vi "诊断标定4.vi"(8 "CAN端口":u16(ring), 9 "设备索引号":u16(ring), 10 "CAN卡类型":u32(ring)=4) -> ()   [LabVIEW 2013] (continued)
                n3552 = local read "设备索引号"() -> (w5173:u16)
                n3553 = local read "CAN卡类型"() -> (w5174:u32)
                n3554 = local read "CAN端口"() -> (w5172:u16)
                n3555 = call "标定授权发送.vi"("CAN卡类型"=w5174, "解锁类型"=enum16{"读取", "写", "下载"}."读取", "设备索引号"=w5173, "CAN端口"=w5172, "是否连接"=TRUE, "板选择"=0, "FUNC"=u32 1) -> ("发送成功"=w5179:bool)  [unwired: 8 out]
              }
            }
            n3556 = case shown="真" w5166 {
              tunnel: w5170 -> [w5181 w5186]
              tunnel: w5169 -> [w5180 w5185]
              tunnel: [w5181 w5183] -> w5168
              tunnel: [w5180 w5182] -> w5167
              frame False {
              }
              frame True {
                n3557 = Enqueue Element(queue=w5186, element="单个读取" ("元素"), error in (no error)=w5185) -> (queue out=w5183:refnum<queue>, error out=w5182:errorcluster)  [unwired: 2 out]
              }
            }
            n3558 = local write "写?"(FALSE ("写?")) -> ()
            n3559 = global write "EV05全局变量1.vi" "输出数组"(u8[] [] ("输出数组")) -> ()
            n3560 = call <vilib>:"Set Busy.vi"("disable click? (T)"=FALSE) -> ()  [unwired: 3 in, 8 out]
            n3561 = local write "清BUFF"(FALSE ("清BUFF")) -> ()
            n3562 = global write "EV05全局变量1.vi" "流控帧 2"(FALSE ("流控帧 2")) -> ()
            n3563 = local write "控制1"(TRUE ("控制1")) -> ()
            n3564 = local write "消除"(TRUE ("消除")) -> ()
          }
        }
      }
      event "全部读取": Value Change {
        n3565 = event-data() -> ("NewVal"=w5191:bool)  [unwired: 5 out]
        n3566 = case shown="真" w5191 {
          tunnel: w5190 -> [w5193 w5197]
          tunnel: w5189 -> [w5192 w5196]
          tunnel: [w5193 w5195] -> w5188
          tunnel: [w5192 w5194] -> w5187
          frame False {
          }
          frame True {
            n3567 = stacked-sequence {
              seq-local: [w5201 _] -> [_ _]
              seq-local: [w5200 _] -> [_ _]
              tunnel: w5197 -> [w5203 w5233]
              tunnel: w5196 -> [w5202 w5232]
              tunnel: [_ w5243] -> w5195
              tunnel: [_ w5242] -> w5194
              frame #0 {
                n3568 = local read "路径"() -> (w5199:path)
                n3569 = Empty String/Path?(string/path=w5199) -> (empty?=w5198:bool)
                n3570 = case shown="假" w5198 {
                  tunnel: w5203 -> [w5212 w5230]
                  tunnel: w5202 -> [w5211 w5229]
                  tunnel: [w5207 w5229] -> w5201
                  tunnel: [w5206 w5230] -> w5200
                  frame False {
                    n3571 = global read "EV05全局变量1.vi" "授权功能"() -> (w5209:bool)
                    n3572 = case shown="假" w5209 {
                      tunnel: [TRUE ("发送成功") w5221] -> w5210
                      frame False {
                      }
                      frame True {
                        n3573 = local read "设备索引号"() -> (w5215:u16)
                        n3574 = local read "CAN卡类型"() -> (w5216:u32)
                        n3575 = local read "CAN端口"() -> (w5214:u16)
                        n3576 = call "标定授权发送.vi"("CAN卡类型"=w5216, "解锁类型"=enum16{"读取", "写", "下载"}."读取", "设备索引号"=w5215, "CAN端口"=w5214, "是否连接"=TRUE, "板选择"=0, "FUNC"=u32 1) -> ("发送成功"=w5221:bool)  [unwired: 8 out]
                      }
                    }
                    n3577 = case shown="真" w5210 {
                      tunnel: w5212 -> [w5223 w5228]
                      tunnel: w5211 -> [w5222 w5227]
                      tunnel: [w5223 w5225] -> w5206
                      tunnel: [w5222 w5224] -> w5207
                      frame False {
                      }
                      frame True {
                        n3578 = Enqueue Element(queue=w5228, element="读配置文件" ("元素"), error in (no error)=w5227) -> (queue out=w5225:refnum<queue>, error out=w5224:errorcluster)  [unwired: 2 out]
                      }
                    }
                    n3579 = call <vilib>:"Set Busy.vi"("disable click? (T)"=FALSE) -> ()  [unwired: 3 in, 8 out]
                    n3580 = local write "布尔"(FALSE ("布尔")) -> ()
                    n3581 = Wait Until Next ms Multiple(millisecond multiple=u32 200 ("毫秒倍数")) -> ()  [unwired: 1 out]
                  }
                  frame True {
                  }
                }
              }
              frame #1 {
                n3582 = global read "EV05全局变量1.vi" "授权功能"() -> (w5236:bool)
                n3583 = case shown="假" w5236 {
                  tunnel: [TRUE ("发送成功") w5252] -> w5241
                  frame False {
                  }
                  frame True {
                    n3584 = local read "设备索引号"() -> (w5246:u16)
                    n3585 = local read "CAN卡类型"() -> (w5247:u32)
                    n3586 = local read "CAN端口"() -> (w5245:u16)
                    n3587 = call "标定授权发送.vi"("CAN卡类型"=w5247, "解锁类型"=enum16{"读取", "写", "下载"}."读取", "设备索引号"=w5246, "CAN端口"=w5245, "是否连接"=TRUE, "板选择"=0, "FUNC"=u32 1) -> ("发送成功"=w5252:bool)  [unwired: 8 out]
                  }
                }
                n3588 = local write "写?"(FALSE ("写?")) -> ()
                n3589 = call <vilib>:"Set Busy.vi"("disable click? (T)"=FALSE) -> ()  [unwired: 3 in, 8 out]
                n3590 = global write "EV05全局变量1.vi" "输出数组"(u8[] [] ("输出数组")) -> ()
                n3591 = global write "EV05全局变量1.vi" "流控帧 2"(FALSE ("流控帧 2")) -> ()
                n3592 = case shown="真" w5241 {
                  tunnel: w5233 -> [w5254 w5259]
                  tunnel: w5232 -> [w5253 w5258]
                  tunnel: [w5254 w5256] -> w5243
                  tunnel: [w5253 w5255] -> w5242
                  frame False {
                  }
                  frame True {
                    n3593 = Enqueue Element(queue=w5259, element="全部读取" ("元素"), error in (no error)=w5258) -> (queue out=w5256:refnum<queue>, error out=w5255:errorcluster)  [unwired: 2 out]
                  }
                }
                n3594 = local write "清BUFF"(FALSE ("清BUFF")) -> ()
                n3595 = local write "控制1"(TRUE ("控制1")) -> ()
                n3596 = local write "消除"(TRUE ("消除")) -> ()
              }
            }
          }
        }
      }
      event "开启均衡": Value Change {
        n3597 = event-data() -> ("NewVal"=w5264:bool)  [unwired: 5 out]
        n3598 = case shown="真" w5264 {
          tunnel: w5263 -> [w5266 w5278]
          tunnel: w5262 -> [w5265 w5277]
          tunnel: [w5266 w5276] -> w5261
          tunnel: [w5265 w5275] -> w5260
          frame False {
          }
          frame True {
            n3599 = global read "EV05全局变量1.vi" "授权功能"() -> (w5270:bool)
            n3600 = case shown="假" w5270 {
              tunnel: [TRUE ("发送成功") w5288] -> w5274
              frame False {
              }
              frame True {
                n3601 = local read "主从选择"() -> (w5280:enum32{"主板", "从板"})
                n3602 = case shown="\"从板\"" w5280 {
                  tunnel: [0.0 ("FUNC") w5290] -> w5281
                  frame "主板", Default {
                  }
                  frame "从板" {
                    n3603 = local read "从板板号"() -> (w5290:u8)
                  }
                }
                n3604 = local read "设备索引号"() -> (w5283:u16)
                n3605 = local read "CAN卡类型"() -> (w5284:u32)
                n3606 = local read "CAN端口"() -> (w5282:u16)
                n3607 = call "标定授权发送.vi"("CAN卡类型"=w5284, "解锁类型"=enum16{"读取", "写", "下载"}."写", "设备索引号"=w5283, "CAN端口"=w5282, "是否连接"=TRUE, "板选择"=0, "FUNC"=w5281) -> ("发送成功"=w5288:bool)  [unwired: 8 out]
              }
            }
            n3608 = case shown="真" w5274 {
              tunnel: w5278 -> [w5292 w5297]
              tunnel: w5277 -> [w5291 w5296]
              tunnel: [w5292 w5294] -> w5276
              tunnel: [w5291 w5293] -> w5275
              frame False {
              }
              frame True {
                n3609 = Enqueue Element(queue=w5297, element="开启均衡" ("元素"), error in (no error)=w5296) -> (queue out=w5294:refnum<queue>, error out=w5293:errorcluster)  [unwired: 2 out]
              }
            }
            n3610 = local write "写?"(TRUE ("写?")) -> ()
            n3611 = local write "清BUFF"(FALSE ("清BUFF")) -> ()
            n3612 = local write "控制1"(TRUE ("控制1")) -> ()
            n3613 = global write "EV05全局变量1.vi" "流控帧 2"(FALSE ("流控帧 2")) -> ()
            n3614 = local write "消除"(TRUE ("消除")) -> ()
            n3615 = call <vilib>:"Set Busy.vi"("disable click? (T)"=TRUE) -> ()  [unwired: 3 in, 8 out]
          }
        }
      }
      event "关闭均衡": Value Change {
        n3616 = event-data() -> ("NewVal"=w5302:bool)  [unwired: 5 out]
        n3617 = case shown="真" w5302 {
          tunnel: w5301 -> [w5304 w5316]
          tunnel: w5300 -> [w5303 w5315]
          tunnel: [w5304 w5314] -> w5299
          tunnel: [w5303 w5313] -> w5298
          frame False {
          }
          frame True {
            n3618 = global read "EV05全局变量1.vi" "授权功能"() -> (w5308:bool)
            n3619 = case shown="假" w5308 {
              tunnel: [TRUE ("发送成功") w5326] -> w5312
              frame False {
              }
              frame True {
                n3620 = local read "主从选择"() -> (w5318:enum32{"主板", "从板"})
                n3621 = case shown="\"从板\"" w5318 {
                  tunnel: [0.0 ("FUNC") w5328] -> w5319
                  frame "主板", Default {
                  }
                  frame "从板" {
                    n3622 = local read "从板板号"() -> (w5328:u8)
                  }
                }
                n3623 = local read "设备索引号"() -> (w5321:u16)
                n3624 = local read "CAN卡类型"() -> (w5322:u32)
                n3625 = local read "CAN端口"() -> (w5320:u16)
                n3626 = call "标定授权发送.vi"("CAN卡类型"=w5322, "解锁类型"=enum16{"读取", "写", "下载"}."写", "设备索引号"=w5321, "CAN端口"=w5320, "是否连接"=TRUE, "板选择"=0, "FUNC"=w5319) -> ("发送成功"=w5326:bool)  [unwired: 8 out]
              }
            }
            n3627 = case shown="真" w5312 {
              tunnel: w5316 -> [w5330 w5335]
              tunnel: w5315 -> [w5329 w5334]
              tunnel: [w5330 w5332] -> w5314
              tunnel: [w5329 w5331] -> w5313
              frame False {
              }
              frame True {
                n3628 = Enqueue Element(queue=w5335, element="关闭均衡" ("元素"), error in (no error)=w5334) -> (queue out=w5332:refnum<queue>, error out=w5331:errorcluster)  [unwired: 2 out]
              }
            }
            n3629 = local write "写?"(TRUE ("写?")) -> ()
            n3630 = local write "清BUFF"(FALSE ("清BUFF")) -> ()
            n3631 = local write "控制1"(TRUE ("控制1")) -> ()
            n3632 = global write "EV05全局变量1.vi" "流控帧 2"(FALSE ("流控帧 2")) -> ()
            n3633 = local write "消除"(TRUE ("消除")) -> ()
            n3634 = call <vilib>:"Set Busy.vi"("disable click? (T)"=TRUE) -> ()  [unwired: 3 in, 8 out]
          }
        }
      }
      event "强制开启均衡": Value Change {
        n3635 = event-data() -> ("NewVal"=w5340:bool)  [unwired: 5 out]
        n3636 = case shown="真" w5340 {
          tunnel: w5339 -> [w5342 w5354]
          tunnel: w5338 -> [w5341 w5353]
          tunnel: [w5342 w5352] -> w5337
          tunnel: [w5341 w5351] -> w5336
          frame False {
          }
          frame True {
            n3637 = global read "EV05全局变量1.vi" "授权功能"() -> (w5346:bool)
            n3638 = case shown="假" w5346 {
              tunnel: [TRUE ("发送成功") w5364] -> w5350
              frame False {
              }
              frame True {
                n3639 = local read "主从选择"() -> (w5356:enum32{"主板", "从板"})
                n3640 = case shown="\"从板\"" w5356 {
                  tunnel: [0.0 ("FUNC") w5366] -> w5357
                  frame "主板", Default {
                  }
                  frame "从板" {
                    n3641 = local read "从板板号"() -> (w5366:u8)
                  }
                }
                n3642 = local read "设备索引号"() -> (w5359:u16)
                n3643 = local read "CAN卡类型"() -> (w5360:u32)
                n3644 = local read "CAN端口"() -> (w5358:u16)
                n3645 = call "标定授权发送.vi"("CAN卡类型"=w5360, "解锁类型"=enum16{"读取", "写", "下载"}."写", "设备索引号"=w5359, "CAN端口"=w5358, "是否连接"=TRUE, "板选择"=0, "FUNC"=w5357) -> ("发送成功"=w5364:bool)  [unwired: 8 out]
              }
            }
            n3646 = case shown="真" w5350 {
              tunnel: w5354 -> [w5368 w5373]
              tunnel: w5353 -> [w5367 w5372]
              tunnel: [w5368 w5370] -> w5352
              tunnel: [w5367 w5369] -> w5351
              frame False {
              }
              frame True {
                n3647 = Enqueue Element(queue=w5373, element="强制均衡" ("元素"), error in (no error)=w5372) -> (queue out=w5370:refnum<queue>, error out=w5369:errorcluster)  [unwired: 2 out]
              }
            }
            n3648 = local write "写?"(TRUE ("写?")) -> ()
            n3649 = local write "清BUFF"(FALSE ("清BUFF")) -> ()
            n3650 = local write "控制1"(TRUE ("控制1")) -> ()
            n3651 = global write "EV05全局变量1.vi" "流控帧 2"(FALSE ("流控帧 2")) -> ()
            n3652 = local write "消除"(TRUE ("消除")) -> ()
            n3653 = call <vilib>:"Set Busy.vi"("disable click? (T)"=TRUE) -> ()  [unwired: 3 in, 8 out]
          }
        }
      }
    }
    n3654 = Unbundle By Name(w2868) -> ("status"=w2867:bool)
    n3655 = Or(x=w2867, y=w2869) -> (x .or. y?=w2870:bool)
  }
  n3656 = while {
    stop <- w5374 stop-if-true
    n3657 = local read "停止"() -> (w5374:bool)
    n3658 = local read "数据读取判定"() -> (w5375:bool)
    n3659 = case shown="真" w5375 {
      frame False {
        n3660 = Wait Until Next ms Multiple(millisecond multiple=u32 50 ("毫秒倍数")) -> ()  [unwired: 1 out]
      }
      frame True {
        n3661 = stacked-sequence {
          frame #0 {
            n3662 = Wait Until Next ms Multiple(millisecond multiple=u32 200 ("毫秒倍数")) -> ()  [unwired: 1 out]
          }
          frame #1 {
            n3663 = local read "临时"() -> (w5381:T1)
            n3664 = Add(x=2, y="循环") -> (x+y=w5379:i32)
            n3665 = for {
              N: w5379 -> [_]
              tunnel: w5381 -> [w5382] mode=indexing
              n3666 = local read "主从选择"() -> (w5383:enum32{"主板", "从板"})
              n3667 = local read "设备索引号"() -> (w5386:u16)
              n3668 = case shown="\"从板\"" w5383 {
                tunnel: [0 ("FUNC") w5392] -> w5384
                frame "主板", Default {
                }
                frame "从板" {
                  n3669 = local read "从板板号"() -> (w5392:u8)
                }
              }
              n3670 = local read "CAN卡类型"() -> (w5385:u32)
              n3671 = local read "CAN端口"() -> (w5387:u16)
              n3672 = local read "选项卡控件 2"() -> (w5390:T6)
              n3673 = disable-structure shown="禁用" {
                disable-tunnel: w5382 -> [w5393 _]
                frame Disabled {
                  n3674 = call "标定授权读取.vi"("VCI_Receive"=w5393) -> ()  [unwired: 1 out]
                }
                frame Enabled {
                }
              }
              n3675 = case shown="\"读写参数\", 默认" w5390 {
                tunnel: "写?" -> [w5400 _ _ _]
                tunnel: "命令" -> [w5401 w5497 w5754 w5886]
                tunnel: w5383 -> [w5408 _ w5760 w5892]
                tunnel: w5382 -> [_ _ _ _]
                tunnel: w5382 -> [w5394 w5488 w5748 w5877]
                tunnel: w5387 -> [w5405 w5498 w5756 w5888]
                tunnel: w5386 -> [w5404 w5499 w5757 w5889]
                tunnel: w5385 -> [w5403 w5500 w5758 w5890]
                tunnel: w5384 -> [w5402 _ w5755 w5887]
                frame "读写参数", Default {
                  n3676 = local read "命令序号"() -> (w5399:u8)
                  n3677 = call "多帧接收机制(EV05).vi"("can卡类型"=w5403, "设备索引号"=w5404, "CAN端口"=w5405, "VCI_Receive"=w5394, "命令"=w5401, "板号"=w5402, "写?"=w5400, "命令序号"=w5399) -> ("错误信号"=w5397:bool, "错误代码"=w5407:i32, "输出数组"=w5406:u8[], "读错误代码"=w5398:u8[], "结束信号"=w5395:bool)  [unwired: 7 out]
                  n3678 = local write "数据读取判定"(FALSE ("数据读取判定")) -> ()
                  n3679 = case shown="假" w5400 {
                    tunnel: w5395 -> [w5418 w5478]
                    tunnel: w5407 -> [w5417 w5477]
                    tunnel: w5399 -> [w5416 _]
                    tunnel: w5406 -> [w5415 _]
                    tunnel: w5401 -> [w5414 _]
                    tunnel: w5408 -> [w5411 w5476]
                    tunnel: w5398 -> [w5410 _]
                    tunnel: w5397 -> [w5409 _]
                    frame False {
                      # "读参数"
                      n3680 = local read "控制1"() -> (w5412:bool)
                      n3681 = And(x=w5412, y=w5418) -> (x .and. y?=w5413:bool)
                      n3682 = case shown="真" w5413 {
                        tunnel: w5417 -> [_ w5428]
                        tunnel: w5416 -> [_ w5427]
                        tunnel: w5415 -> [_ w5426]
                        tunnel: w5414 -> [_ w5425]
                        tunnel: w5411 -> [_ w5422]
                        tunnel: w5410 -> [_ w5420]
                        tunnel: w5409 -> [_ w5421]
                        frame False {
                        }
                        frame True {
                          n3683 = case shown="假" w5421 {
                            tunnel: w5428 -> [w5437 _]
                            tunnel: w5427 -> [w5436 _]
                            tunnel: w5426 -> [w5435 _]
                            tunnel: w5425 -> [w5433 _]
                            tunnel: w5422 -> [w5429 _]
                            tunnel: w5420 -> [_ w5462]
                            frame False {
                              n3684 = case shown="\"主板\", 默认" w5429 {
                                tunnel: [w5438 _] -> w5432
                                tunnel: [_ w5451] -> w5431
                                frame "主板", Default {
                                n3685 = stacked-sequence {
                                tunnel: [_ w5450] -> w5438
                                frame #0 {
                                n3686 = control-ref of="一级故障"() -> (w5444:refnum<vi>)
                                n3687 = control-ref of="一级故障 2"() -> (w5446:refnum<vi>)
                                n3688 = control-ref of="一级故障 3"() -> (w5447:refnum<vi>)
                                n3689 = control-ref of="加热控制参数"() -> (w5448:refnum<vi>)
                                n3690 = control-ref of="充电控制参数"() -> (w5449:refnum<vi>)
                                n3691 = control-ref of="电池信息"() -> (w5442:refnum<vi>)
                                n3692 = control-ref of="项目信息"() -> (w5445:refnum<vi>)
                                n3693 = control-ref of="一级故障 4"() -> (w5443:refnum<vi>)
                                n3694 = control-ref of="高压参数"() -> (w5441:refnum<vi>)
                                n3695 = local read "主板数据"() -> (w5440:T4)
                                n3696 = Bundle(cluster=w5440, "项目信息"=w5445, "一级故障 4"=w5443, "一级故障"=w5444, "一级故障 2"=w5446, "一级故障 3"=w5447, "加热控制参数"=w5448, "充电控制参数"=w5449, "高压参数"=w5441, "电池信息"=w5442) -> (w5439:T4)
                                n3697 = local write "主板数据"(w5439) -> ()
                                }
                                frame #1 {
                                n3698 = control-ref of="主板数据"() -> (w5450:refnum<vi>)
                                }
                                }
                                }
                                frame "从板" {
                                n3699 = stacked-sequence {
                                tunnel: [_ w5461] -> w5451
                                frame #0 {
                                n3700 = control-ref of="从板板号"() -> (w5454:refnum<vi>)
                                n3701 = control-ref of="项目信息 2"() -> (w5455:refnum<vi>)
                                n3702 = control-ref of="加热控制参数"() -> (w5456:refnum<vi>)
                                n3703 = control-ref of="一级故障(从板)"() -> (w5457:refnum<vi>)
                                n3704 = control-ref of="二级故障(从板)"() -> (w5458:refnum<vi>)
                                n3705 = control-ref of="三级故障(从板)"() -> (w5459:refnum<vi>)
                                n3706 = control-ref of="电池组信息(从板)"() -> (w5460:refnum<vi>)
                                n3707 = local read "从板数据"() -> (w5453:T3)
                                n3708 = Bundle(cluster=w5453, "从板板号"=w5454, "项目信息 2"=w5455, "加热控制参数"=w5456, "一级故障(从板)"=w5457, "二级故障(从板)"=w5458, "三级故障(从板)"=w5459, "电池组信息(从板)"=w5460) -> (w5452:T3)
                                n3709 = local write "从板数据"(w5452) -> ()
                                }
                                frame #1 {
                                n3710 = control-ref of="从板数据"() -> (w5461:refnum<vi>)
                                }
                                }
                                }
                              }
                              n3711 = control-ref of="结果"() -> (w5434:refnum<vi>)
                              n3712 = control-ref of="从板个数"() -> (w5430:refnum<vi>)
                              n3713 = call "输出数据解析.vi"("主板引用"=w5432, "从板引用"=w5431, "板选择"=w5429, "错误代码"=w5437, "命令序号"=w5436, "输入数组"=w5435, "命令"=w5433, "进度引用"=w5434, "从板个数"=w5430) -> ()  [unwired: 7 out]
                            }
                            frame True {
                              n3714 = Index Array(array=w5462, index #1=0 ("索引"), index #2=1 ("索引")) -> (element #1=w5465:u8, element #2=w5466:u8)
                              n3715 = Join Numbers(hi=w5465, lo=w5466) -> ((hi.lo)=w5464:u16)
                              n3716 = Number To Hexadecimal String(2:w5464) -> (0:w5463:string)  [unwired: 1 out]
                              n3717 = control-ref of="结果"() -> (w5471:refnum<vi>)
                              n3718 = Concatenate Strings("0x" ("字符串"), w5463) -> (w5472:string)
                              n3719 = Build Array(w5472) -> (w5473:string[])
                              n3720 = call "表格编辑.vi"("新元素/子数组"=w5473, "活动单元格:单元格背景色"=u32 16740749, "MCListbox引用句柄"=w5471) -> ()  [unwired: 9 out]
                            }
                          }
                          n3721 = global write "EV05全局变量1.vi" "流控帧 2"(FALSE ("流控帧 2")) -> ()
                          n3722 = local write "消除"(FALSE ("消除")) -> ()
                          n3723 = local write "控制1"(FALSE ("控制1")) -> ()
                        }
                      }
                    }
                    frame True {
                      # "写参数判定"
                      n3724 = And(x="控制1", y=w5478) -> (x .and. y?=w5475:bool)
                      n3725 = case shown="真" w5475 {
                        tunnel: w5477 -> [_ w5485]
                        tunnel: w5476 -> [_ w5482]
                        frame False {
                        }
                        frame True {
                          n3726 = call <vilib>:"Unset Busy.vi"() -> ()  [unwired: 2 in, 10 out]
                          n3727 = case shown="\"主板\", 默认" w5482 {
                            tunnel: [w5486 w5487] -> w5484
                            frame "主板", Default {
                              n3728 = local read "主板选项"() -> (w5486:string)
                            }
                            frame "从板" {
                              n3729 = local read "从板选项"() -> (w5487:string)
                            }
                          }
                          n3730 = control-ref of="结果"() -> (w5483:refnum<vi>)
                          n3731 = call "输入数据判定.vi"("主从选择"=w5482, "主板选项"=w5484, "进度引用"=w5483, "错误代码"=w5485) -> ()  [unwired: 2 in, 6 out]
                          n3732 = global write "EV05全局变量1.vi" "流控帧 2"(FALSE ("流控帧 2")) -> ()
                          n3733 = local write "控制1"(FALSE ("控制1")) -> ()
                          n3734 = local write "消除"(FALSE ("消除")) -> ()
                        }
                      }
                    }
                  }
                }
                frame "版本读取" {
                  n3735 = local read "命令序号"() -> (w5491:u8)
                  n3736 = local read "从板板号"() -> (w5494:u8)
                  n3737 = local read "控制1"() -> (w5495:bool)
                  n3738 = call "多帧接收机制(EV05).vi"("can卡类型"=w5500, "设备索引号"=w5499, "CAN端口"=w5498, "VCI_Receive"=w5488, "命令"=w5497, "板号"=w5494, "命令序号"=w5491) -> ("错误信号"=w5492:bool, "输出数组"=w5501:u8[], "读错误代码"=w5493:u8[], "结束信号"=w5489:bool)  [unwired: 1 in, 8 out]
                  n3739 = And(x=w5495, y=w5489) -> (x .and. y?=w5496:bool)
                  n3740 = case shown="真" w5496 {
                    tunnel: w5501 -> [_ w5509]
                    tunnel: w5491 -> [_ w5508]
                    tunnel: w5497 -> [_ w5507]
                    tunnel: w5493 -> [_ w5503]
                    tunnel: w5492 -> [_ w5502]
                    frame False {
                    }
                    frame True {
                      n3741 = case shown="假" w5502 {
                        tunnel: w5509 -> [w5513 _]
                        tunnel: w5508 -> [w5512 _]
                        tunnel: w5507 -> [w5511 _]
                        tunnel: w5503 -> [w5510 w5737]
                        frame False {
                          n3742 = case shown="89" w5511 {
                            tunnel: w5512 -> [_ w5516]
                            tunnel: w5513 -> [_ w5515]
                            tunnel: w5510 -> [_ _]
                            frame 0, Default {
                            }
                            frame 137 {
                              n3743 = case shown="1" w5516 {
                                tunnel: w5515 -> [_ w5544 w5588 w5608 w5735]
                                frame 0, Default {
                                }
                                frame 1 {
                                w5526 = "." ("字符串")
                                n3744 = Array Subset(array=w5544, index=0 ("索引"), length=14 ("长度")) -> (w5557:u8[])
                                n3745 = Index Array(array=w5544, index=14 ("索引")) -> (element=w5547:u8)
                                n3746 = Index Array(array=w5544, index #1=15 ("索引"), index #2=16 ("索引")) -> (element #1=w5553:u8, element #2=w5554:u8)
                                n3747 = Index Array(array=w5544, index #1=17 ("索引"), index #2=18 ("索引")) -> (element #1=w5548:u8, element #2=w5549:u8)
                                n3748 = call "数组去零.vi"("输入"=w5557) -> ("输出"=w5532:dbl[])
                                n3749 = Join Numbers(hi=w5548, lo=w5549) -> ((hi.lo)=w5545:u16)
                                n3750 = Join Numbers(hi=w5553, lo=w5554) -> ((hi.lo)=w5546:u16)
                                n3751 = Number To Decimal String(number=w5547) -> (decimal integer string=w5539:string)  [unwired: 1 out]
                                n3752 = Byte Array To String(unsigned byte array=w5532) -> (string=w5531:string)
                                n3753 = Number To Decimal String(number=w5545) -> (decimal integer string=w5527:string)  [unwired: 1 out]
                                n3754 = Number To Decimal String(number=w5546) -> (decimal integer string=w5538:string)  [unwired: 1 out]
                                n3755 = Array Subset(array=w5544, index=21 ("索引"), length=7 ("长度")) -> (w5541:u8[])
                                n3756 = Concatenate Strings("V" ("字符串"), w5539, w5526, w5538, w5526, w5527) -> (w5536:string)
                                n3757 = call "数组去零.vi"("输入"=w5541) -> ("输出"=w5524:dbl[])
                                n3758 = Byte Array To String(unsigned byte array=w5524) -> (string=w5522:string)
                                n3759 = call <vilib>:"Space Constant.vi"() -> ("String"=w5523:string)
                                n3760 = Equal?(x=w5522, y=w5523) -> (x = y?=w5528:bool)
                                n3761 = Concatenate Strings("-" ("字符串"), w5522) -> (w5529:string)
                                n3762 = Select(t=w5523, s=w5528, f=w5529) -> (s? t:f=w5525:string)
                                n3763 = Concatenate Strings(w5531, "-" ("字符串"), w5536, w5525) -> (w5518:string)
                                n3764 = local read "项目软件版本"() -> (w5520:string[])
                                n3765 = local read "从板板号"() -> (w5517:u8)
                                n3766 = local write "项目软件版本号"(w5518) -> ()
                                n3767 = Replace Array Subset(array=w5520, new element=w5518, index=w5517) -> (w5519:string[])
                                n3768 = control-ref of="结果"() -> (w5535:refnum<vi>)
                                n3769 = local write "项目软件版本"(w5519) -> ()
                                n3770 = Build Array("项目软件版本     读取完成" ("读取结果")) -> (w5533:string[])
                                n3771 = call "表格编辑(版本读取).vi"("新元素/子数组"=w5533, "活动单元格:单元格背景色"=u32 6618880, "MCListbox引用句柄"=w5535) -> ()  [unwired: 9 out]
                                }
                                frame 2 {
                                w5571 = ""
                                w5568 = "." ("字符串")
                                n3772 = Array Subset(array=w5588, index=0 ("索引"), length=14 ("长度")) -> (w5576:u8[])
                                n3773 = Index Array(array=w5588, index=14 ("索引")) -> (element=w5591:u8)
                                n3774 = Index Array(array=w5588, index #1=15 ("索引"), index #2=16 ("索引")) -> (element #1=w5597:u8, element #2=w5598:u8)
                                n3775 = Index Array(array=w5588, index #1=17 ("索引"), index #2=18 ("索引")) -> (element #1=w5592:u8, element #2=w5593:u8)
                                n3776 = Join Numbers(hi=w5592, lo=w5593) -> ((hi.lo)=w5589:u16)
                                n3777 = Join Numbers(hi=w5597, lo=w5598) -> ((hi.lo)=w5590:u16)
                                n3778 = Number To Decimal String(number=w5589) -> (decimal integer string=w5569:string)  [unwired: 1 out]
                                n3779 = call "数组去零.vi"("输入"=w5576) -> ("输出"=w5575:dbl[])
                                n3780 = Number To Decimal String(number=w5591) -> (decimal integer string=w5583:string)  [unwired: 1 out]
                                n3781 = Number To Decimal String(number=w5590) -> (decimal integer string=w5582:string)  [unwired: 1 out]
                                n3782 = Array Subset(array=w5588, index=21 ("索引"), length=7 ("长度")) -> (w5585:u8[])
                                n3783 = Byte Array To String(unsigned byte array=w5575) -> (string=w5570:string)
                                n3784 = call "数组去零.vi"("输入"=w5585) -> ("输出"=w5567:dbl[])
                                n3785 = Concatenate Strings("V" ("字符串"), w5583, w5568, w5582, w5568, w5569) -> (w5580:string)
                                n3786 = Byte Array To String(unsigned byte array=w5567) -> (string=w5565:string)
                                n3787 = Equal?(x=w5571, y=w5565) -> (x = y?=w5572:bool)
                                n3788 = Concatenate Strings("-" ("字符串"), w5565) -> (w5573:string)
                                n3789 = Select(t=w5571, s=w5572, f=w5573) -> (s? t:f=w5566:string)
                                n3790 = Concatenate Strings(w5570, "-" ("字符串"), w5580, w5566) -> (w5561:string)
                                n3791 = local read "平台软件版本"() -> (w5563:string[])
                                n3792 = local read "从板板号"() -> (w5560:u8)
                                n3793 = local write "平台软件版本号"(w5561) -> ()
                                n3794 = Replace Array Subset(array=w5563, new element=w5561, index=w5560) -> (w5562:string[])
                                n3795 = control-ref of="结果"() -> (w5578:refnum<vi>)
                                n3796 = local write "平台软件版本"(w5562) -> ()
                                n3797 = Build Array("平台软件版本     读取完成" ("读取结果")) -> (w5577:string[])
                                n3798 = call "表格编辑(版本读取).vi"("新元素/子数组"=w5577, "活动单元格:单元格背景色"=u32 6618880, "MCListbox引用句柄"=w5578) -> ()  [unwired: 1 in, 8 out]
                                }
                                frame 3 {
                                n3799 = Index Array(array=w5608, index #1=0 ("索引"), index #2=1 ("索引")) -> (element #1=w5604:u8, element #2=w5605:u8)
                                n3800 = Join Numbers(hi=w5604, lo=w5605) -> ((hi.lo)=w5603:u16)
                                n3801 = case shown="99, 默认" w5603 {
                                tunnel: w5608 -> [w5611 _ w5645]
                                tunnel: w5603 -> [_ _ w5623]
                                frame 0 {
                                n3802 = Index Array(array=w5611, index #1=2 ("索引"), index #2=3 ("索引")) -> (element #1=w5615:u8, element #2=w5614:u8)
                                n3803 = Join Numbers(hi=w5615, lo=w5614) -> ((hi.lo)=w5610:u16)
                                n3804 = for {
                                N: w5610 -> [_]
                                tunnel: w5611 -> [w5620]
                                tunnel: [w5616] -> w5609 mode=indexing
                                i -> [w5619]
                                n3805 = Add(x=w5619, y=4) -> (x+y=w5617:i32)
                                n3806 = Index Array(array=w5620, index=w5617) -> (element=w5616:u8)
                                }
                                "MODEL号" <- w5609
                                }
                                frame 99, Default {
                                }
                                frame 1..40 {
                                w5628 = ""
                                w5649 = "." ("字符串")
                                n3807 = Array Subset(array=w5645, index=2 ("索引"), length=14 ("长度")) -> (w5634:u8[])
                                n3808 = Index Array(array=w5645, index=16 ("索引")) -> (element=w5657:u8)
                                n3809 = Index Array(array=w5645, index #1=17 ("索引"), index #2=18 ("索引")) -> (element #1=w5663:u8, element #2=w5664:u8)
                                n3810 = Index Array(array=w5645, index #1=19 ("索引"), index #2=20 ("索引")) -> (element #1=w5658:u8, element #2=w5659:u8)
                                n3811 = Join Numbers(hi=w5658, lo=w5659) -> ((hi.lo)=w5655:u16)
                                n3812 = Join Numbers(hi=w5663, lo=w5664) -> ((hi.lo)=w5656:u16)
                                n3813 = Number To Decimal String(number=w5623) -> (decimal integer string=w5643:string)  [unwired: 1 out]
                                n3814 = Number To Decimal String(number=w5657) -> (decimal integer string=w5651:string)  [unwired: 1 out]
                                n3815 = call "数组去零.vi"("输入"=w5634) -> ("输出"=w5633:dbl[])
                                n3816 = Number To Decimal String(number=w5656) -> (decimal integer string=w5650:string)  [unwired: 1 out]
                                n3817 = Number To Decimal String(number=w5655) -> (decimal integer string=w5648:string)  [unwired: 1 out]
                                n3818 = Byte Array To String(unsigned byte array=w5633) -> (string=w5635:string)
                                n3819 = Concatenate Strings("第" ("读取结果"), w5643, "模块" ("字符串"), "     读取完成" ("读取结果")) -> (w5636:string)
                                n3820 = Concatenate Strings("V" ("字符串"), w5651, w5649, w5650, w5649, w5648) -> (w5646:string)
                                n3821 = control-ref of="结果"() -> (w5639:refnum<vi>)
                                n3822 = Array Subset(array=w5645, index=23 ("索引"), length=7 ("长度")) -> (w5632:u8[])
                                n3823 = call "数组去零.vi"("输入"=w5632) -> ("输出"=w5627:dbl[])
                                n3824 = Byte Array To String(unsigned byte array=w5627) -> (string=w5624:string)
                                n3825 = Build Array(w5636) -> (w5638:string[])
                                n3826 = control-ref of="模块软件版本"() -> (w5640:refnum<vi>)
                                n3827 = local read "模块软件版本"() -> (w5641:T16)
                                n3828 = Equal?(x=w5628, y=w5624) -> (x = y?=w5629:bool)
                                n3829 = call "表格编辑(版本读取).vi"("新元素/子数组"=w5638, "活动单元格:单元格背景色"=u32 6618880, "MCListbox引用句柄"=w5639) -> ()  [unwired: 1 in, 8 out]
                                n3830 = Concatenate Strings("-" ("字符串"), w5624) -> (w5630:string)
                                n3831 = Select(t=w5628, s=w5629, f=w5630) -> (s? t:f=w5626:string)
                                n3832 = Concatenate Strings(w5635, "-" ("字符串"), w5646, w5626) -> (w5625:string)
                                n3833 = case shown="30" w5623 {
                                tunnel: [_ "VERSIONM" "BCUMCAL" "BMUMCAL" "BMURMCAL" "BCUCMCAL" "BCUDMCAL" "SCH" "BSW" "CDD" "DATALAYER" "DATAANALYSIS" "SOC" "SOH" "SOF" "INTRES" "INTCAN" "CARCAN" "CHGCANL" "THM" "CHGM" "HVM" "LVM" "BALM" "SAFEM" "RUNMODEM" "RELAY" "DO" "GBCHGDET" "SUPPLYPOWGDET" "SUMVDET" "CURDET" "TEMPERDET" "CELLVDET" "ISODET" "AI" "DI" "SYSCONF" "ECUCONF"] -> w5622
                                frame 0, Default {
                                }
                                frame 1 {
                                }
                                frame 2 {
                                }
                                frame 3 {
                                }
                                frame 4 {
                                }
                                frame 5 {
                                }
                                frame 6 {
                                }
                                frame 7 {
                                }
                                frame 8 {
                                }
                                frame 9 {
                                }
                                frame 10 {
                                }
                                frame 11 {
                                }
                                frame 12 {
                                }
                                frame 13 {
                                }
                                frame 14 {
                                }
                                frame 15 {
                                }
                                frame 16 {
                                }
                                frame 17 {
                                }
                                frame 18 {
                                }
                                frame 19 {
                                }
                                frame 20 {
                                }
                                frame 21 {
                                }
                                frame 22 {
                                }
                                frame 23 {
                                }
                                frame 24 {
                                }
                                frame 25 {
                                }
                                frame 26 {
                                }
                                frame 27 {
                                }
                                frame 28 {
                                }
                                frame 29 {
                                }
                                frame 30 {
                                }
                                frame 31 {
                                }
                                frame 32 {
                                }
                                frame 33 {
                                }
                                frame 34 {
                                }
                                frame 35 {
                                }
                                frame 36 {
                                }
                                frame 37 {
                                }
                                frame 38 {
                                }
                                }
                                n3834 = case shown="\"全部读取\"" w5641 {
                                tunnel: w5625 -> [w5708 w5716]
                                tunnel: w5623 -> [w5712 w5721]
                                tunnel: w5640 -> [w5714 w5722]
                                tunnel: w5622 -> [w5713 w5720]
                                frame "全部读取" {
                                n3835 = Number To Decimal String(number=w5712) -> (decimal integer string=w5711:string)  [unwired: 1 out]
                                n3836 = Concatenate Strings(w5711, "-" ("元素"), w5713) -> (w5709:string)
                                n3837 = Build Array(w5709, w5708) -> (w5707:string[])
                                n3838 = call "表格编辑(模块版本).vi"("新元素/子数组"=w5707, "MCListbox引用句柄"=w5714) -> ()  [unwired: 1 in, 9 out]
                                }
                                frame "BCUMCAL", Default {
                                n3839 = Number To Decimal String(number=w5721) -> (decimal integer string=w5719:string)  [unwired: 1 out]
                                n3840 = Concatenate Strings(w5719, "-" ("元素"), w5720) -> (w5717:string)
                                n3841 = Build Array(w5717, w5716) -> (w5715:string[])
                                n3842 = call "表格编辑(模块版本).vi"("新元素/子数组"=w5715, "MCListbox引用句柄"=w5722) -> ()  [unwired: 1 in, 9 out]
                                }
                                }
                                }
                                }
                                }
                                frame 4 {
                                n3843 = Array Subset(array=w5735, length=12 ("长度")) -> (w5733:u8[])  [unwired: 1 in]
                                n3844 = Byte Array To String(unsigned byte array=w5733) -> (string=w5732:string)
                                n3845 = call <vilib>:"Trim Whitespace.vi"("string"=w5732) -> ("trimmed string"=w5724:string)  [unwired: 1 in]
                                n3846 = local read "从板板号"() -> (w5723:u8)
                                n3847 = local write "硬件版本号"(w5724) -> ()
                                n3848 = local read "硬件版本"() -> (w5725:string[])
                                n3849 = Replace Array Subset(array=w5725, new element=w5724, index=w5723) -> (w5726:string[])
                                n3850 = local write "硬件版本"(w5726) -> ()
                                n3851 = global write "EV05全局变量1.vi" "写入超时"(TRUE ("写入超时")) -> ()
                                n3852 = control-ref of="结果"() -> (w5730:refnum<vi>)
                                n3853 = Build Array("硬件版本     读取完成" ("读取结果")) -> (w5729:string[])
                                n3854 = call "表格编辑(版本读取).vi"("新元素/子数组"=w5729, "活动单元格:单元格背景色"=u32 6618880, "MCListbox引用句柄"=w5730) -> ()  [unwired: 9 out]
                                }
                              }
                              n3855 = global write "EV05全局变量1.vi" "写入超时"(TRUE ("写入超时")) -> ()
                            }
                          }
                        }
                        frame True {
                          n3856 = Index Array(array=w5737, index #1=0 ("索引"), index #2=1 ("索引")) -> (element #1=w5742:u8, element #2=w5743:u8)
                          n3857 = Join Numbers(hi=w5742, lo=w5743) -> ((hi.lo)=w5741:u16)
                          n3858 = Number To Hexadecimal String(2:w5741) -> (0:w5740:string)  [unwired: 1 out]
                          n3859 = control-ref of="结果"() -> (w5739:refnum<vi>)
                          n3860 = Concatenate Strings("0x" ("字符串"), w5740) -> (w5747:string)
                          n3861 = Build Array(w5747) -> (w5738:string[])
                          n3862 = call "表格编辑(版本读取).vi"("新元素/子数组"=w5738, "活动单元格:单元格背景色"=u32 16740749, "MCListbox引用句柄"=w5739) -> ()  [unwired: 9 out]
                        }
                      }
                      n3863 = global write "EV05全局变量1.vi" "流控帧 2"(FALSE ("流控帧 2")) -> ()
                      n3864 = local write "控制1"(FALSE ("控制1")) -> ()
                      n3865 = local write "消除"(FALSE ("消除")) -> ()
                      n3866 = call <vilib>:"Unset Busy.vi"() -> ()  [unwired: 2 in, 10 out]
                    }
                  }
                  n3867 = local write "数据读取判定"(FALSE ("数据读取判定")) -> ()
                }
                frame "其它诊断" {
                  n3868 = local read "命令序号"() -> (w5752:u8)
                  n3869 = call "多帧接收机制(EV05).vi"("can卡类型"=w5758, "设备索引号"=w5757, "CAN端口"=w5756, "VCI_Receive"=w5748, "命令"=w5754, "板号"=w5755, "命令序号"=w5752) -> ("错误代码"=w5759:i32, "输出数组"=w5753:u8[], "读错误代码"=w5751:u8[], "结束信号"=w5749:bool)  [unwired: 1 in, 8 out]
                  n3870 = case shown="真" w5749 {
                    tunnel: w5760 -> [_ w5761]
                    tunnel: w5759 -> [_ _]
                    tunnel: w5753 -> [_ w5762]
                    tunnel: w5752 -> [_ w5765]
                    tunnel: w5751 -> [_ w5763]
                    frame False {
                    }
                    frame True {
                      n3871 = Insert Into Array(array=w5763, new element=w5762) -> (w5764:u8[])  [unwired: 1 in]
                      n3872 = case shown="2" w5765 {
                        tunnel: w5764 -> [_ w5774 w5851]
                        tunnel: w5761 -> [_ _ w5846]
                        frame 0, Default {
                        }
                        frame 1 {
                          n3873 = Index Array(array=w5774) -> (element #1=w5773:u8, element #2=w5772:u8, element #3=w5771:u8)  [unwired: 3 in]
                          n3874 = Join Numbers(hi=w5772, lo=w5771) -> ((hi.lo)=w5770:u16)
                          n3875 = case shown="1" w5773 {
                            tunnel: w5774 -> [_ _ _ _ _ _ _ _ _]
                            tunnel: w5770 -> [_ w5777 w5784 w5793 w5802 w5811 w5820 w5829 w5838]
                            frame 0, Default {
                              n3876 = local write "继电器超时处理"(FALSE ("继电器超时处理")) -> ()
                            }
                            frame 1 {
                              n3877 = Equal To 0?(x=w5777) -> (x = 0?=w5776:bool)
                              n3878 = local write "正级继电器 12"(w5776) -> ()
                              n3879 = case shown="假" w5776 {
                                tunnel: w5777 -> [w5779 _]
                                frame False {
                                n3880 = local read "正级继电器"() -> (w5781:bool)
                                n3881 = Number To Hexadecimal String(2:w5779) -> (0:w5778:string)  [unwired: 1 out]
                                n3882 = Not(x=w5781) -> (.not. x?=w5780:bool)
                                n3883 = Concatenate Strings("继电器操作失败,0x" ("消息"), w5778) -> ()  [unwired: 1 out]
                                n3884 = local write "正级继电器"(w5780) -> ()
                                }
                                frame True {
                                (unwired) "继电器操作成功!\n继电器操作成功!\n继电器操作成功!"
                                }
                              }
                            }
                            frame 2 {
                              n3885 = Equal To 0?(x=w5784) -> (x = 0?=w5783:bool)
                              n3886 = local write "正级继电器 2"(w5783) -> ()
                              n3887 = case shown="假" w5783 {
                                tunnel: w5784 -> [w5789 _]
                                tunnel: [w5787 "继电器操作成功!\n继电器操作成功!\n继电器操作成功!"] -> _
                                frame False {
                                n3888 = local read "负级继电器"() -> (w5785:bool)
                                n3889 = Number To Hexadecimal String(2:w5789) -> (0:w5788:string)  [unwired: 1 out]
                                n3890 = Not(x=w5785) -> (.not. x?=w5786:bool)
                                n3891 = Concatenate Strings("继电器操作失败,0x" ("消息"), w5788) -> (w5787:string)
                                n3892 = local write "负级继电器"(w5786) -> ()
                                }
                                frame True {
                                }
                              }
                            }
                            frame 3 {
                              n3893 = Equal To 0?(x=w5793) -> (x = 0?=w5792:bool)
                              n3894 = case shown="假" w5792 {
                                tunnel: w5793 -> [w5798 _]
                                tunnel: [w5796 "继电器操作成功!\n继电器操作成功!\n继电器操作成功!"] -> _
                                frame False {
                                n3895 = local read "预充电继电器"() -> (w5794:bool)
                                n3896 = Number To Hexadecimal String(2:w5798) -> (0:w5797:string)  [unwired: 1 out]
                                n3897 = Not(x=w5794) -> (.not. x?=w5795:bool)
                                n3898 = Concatenate Strings("继电器操作失败,0x" ("消息"), w5797) -> (w5796:string)
                                n3899 = local write "预充电继电器"(w5795) -> ()
                                }
                                frame True {
                                }
                              }
                              n3900 = local write "正级继电器 3"(w5792) -> ()
                            }
                            frame 4 {
                              n3901 = Equal To 0?(x=w5802) -> (x = 0?=w5801:bool)
                              n3902 = case shown="假" w5801 {
                                tunnel: w5802 -> [w5807 _]
                                tunnel: [w5805 "继电器操作成功!\n继电器操作成功!\n继电器操作成功!"] -> _
                                frame False {
                                n3903 = local read "加热继电器"() -> (w5804:bool)
                                n3904 = Number To Hexadecimal String(2:w5807) -> (0:w5806:string)  [unwired: 1 out]
                                n3905 = Not(x=w5804) -> (.not. x?=w5803:bool)
                                n3906 = Concatenate Strings("继电器操作失败,0x" ("消息"), w5806) -> (w5805:string)
                                n3907 = local write "加热继电器"(w5803) -> ()
                                }
                                frame True {
                                }
                              }
                              n3908 = local write "正级继电器 5"(w5801) -> ()
                            }
                            frame 5 {
                              n3909 = Equal To 0?(x=w5811) -> (x = 0?=w5810:bool)
                              n3910 = case shown="假" w5810 {
                                tunnel: w5811 -> [w5816 _]
                                tunnel: [w5814 "继电器操作成功!\n继电器操作成功!\n继电器操作成功!"] -> _
                                frame False {
                                n3911 = local read "充电继电器"() -> (w5812:bool)
                                n3912 = Number To Hexadecimal String(2:w5816) -> (0:w5815:string)  [unwired: 1 out]
                                n3913 = Not(x=w5812) -> (.not. x?=w5813:bool)
                                n3914 = Concatenate Strings("继电器操作失败,0x" ("消息"), w5815) -> (w5814:string)
                                n3915 = local write "充电继电器"(w5813) -> ()
                                }
                                frame True {
                                }
                              }
                              n3916 = local write "正级继电器 4"(w5810) -> ()
                            }
                            frame 6 {
                              n3917 = Equal To 0?(x=w5820) -> (x = 0?=w5819:bool)
                              n3918 = local write "正级继电器 6"(w5819) -> ()
                              n3919 = case shown="假" w5819 {
                                tunnel: w5820 -> [w5825 _]
                                tunnel: [w5823 "继电器操作成功!\n继电器操作成功!\n继电器操作成功!"] -> _
                                frame False {
                                n3920 = local read "风机继电器"() -> (w5821:bool)
                                n3921 = Number To Hexadecimal String(2:w5825) -> (0:w5824:string)  [unwired: 1 out]
                                n3922 = Not(x=w5821) -> (.not. x?=w5822:bool)
                                n3923 = Concatenate Strings("继电器操作失败,0x" ("消息"), w5824) -> (w5823:string)
                                n3924 = local write "风机继电器"(w5822) -> ()
                                }
                                frame True {
                                }
                              }
                            }
                            frame 7 {
                              n3925 = Equal To 0?(x=w5829) -> (x = 0?=w5828:bool)
                              n3926 = case shown="假" w5828 {
                                tunnel: w5829 -> [w5834 _]
                                tunnel: [w5832 "继电器操作成功!\n继电器操作成功!\n继电器操作成功!"] -> _
                                frame False {
                                n3927 = local read "加热继电器"() -> (w5830:bool)
                                n3928 = Number To Hexadecimal String(2:w5834) -> (0:w5833:string)  [unwired: 1 out]
                                n3929 = Not(x=w5830) -> (.not. x?=w5831:bool)
                                n3930 = Concatenate Strings("继电器操作失败,0x" ("消息"), w5833) -> (w5832:string)
                                n3931 = local write "加热继电器"(w5831) -> ()
                                }
                                frame True {
                                }
                              }
                              n3932 = local write "正级继电器 7"(w5828) -> ()
                            }
                            frame 8 {
                              n3933 = Equal To 0?(x=w5838) -> (x = 0?=w5837:bool)
                              n3934 = case shown="假" w5837 {
                                tunnel: w5838 -> [w5843 _]
                                tunnel: [w5841 "继电器操作成功!\n继电器操作成功!\n继电器操作成功!"] -> _
                                frame False {
                                n3935 = local read "风机继电器"() -> (w5839:bool)
                                n3936 = Number To Hexadecimal String(2:w5843) -> (0:w5842:string)  [unwired: 1 out]
                                n3937 = Not(x=w5839) -> (.not. x?=w5840:bool)
                                n3938 = Concatenate Strings("继电器操作失败,0x" ("消息"), w5842) -> (w5841:string)
                                n3939 = local write "风机继电器"(w5840) -> ()
                                }
